vi "ref_MCListbox_call.vi"(8 "VI引用输入":refnum<vi>, 9 "清除原有数据":bool, 10 "数组":string[][](array[string])) -> ()   [LabVIEW 2016]
uses:
  <vilib>/Utility/miscctls.llb/LVRowAndColumnTypeDef.ctl
  Global Variables/Pacemaker ASIC Test_Save_SN Globals.vi
  Global Variables/Pacemaker ASIC Test_Config Globals.vi
  <vilib>/Utility/file.llb/Write Delimited Spreadsheet (string).vi
panel:
  out "数组 2":string[](array[string])
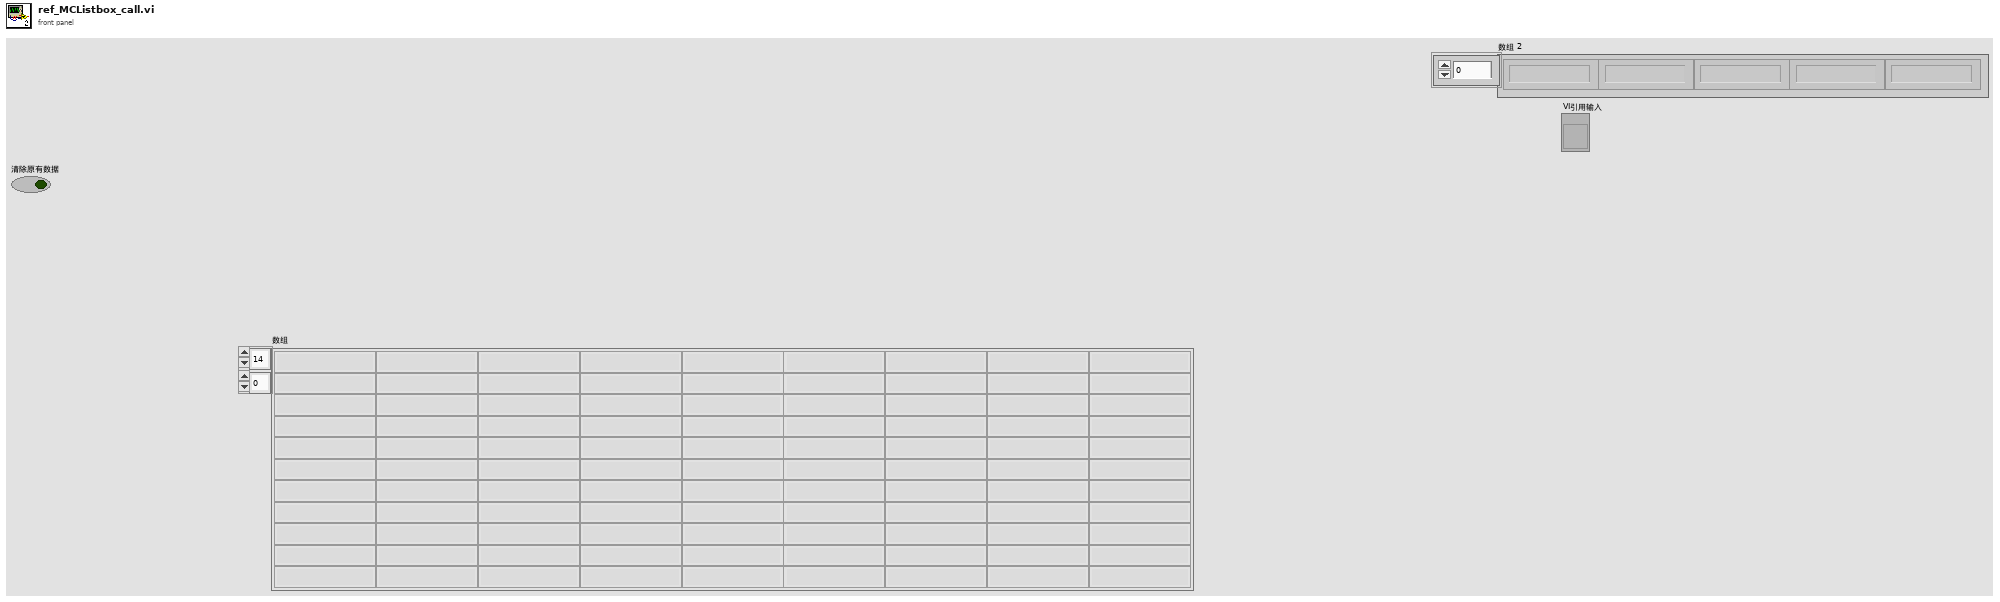
[diagram p1: front panel]
types:
  T1 = cluster{"LED1":refnum<vi>, "LED2":refnum<vi>, "LED3":refnum<vi>, "LED4":refnum<vi>, "LED5":refnum<vi>, "LED7":refnum<vi>, "LED8":refnum<vi>, "LED9":refnum<vi>, "LED10":refnum<vi>}
  T2 = typedef "LVRowAndColumnTypeDef.ctl" = cluster{"Row":i32, "Column":i32}
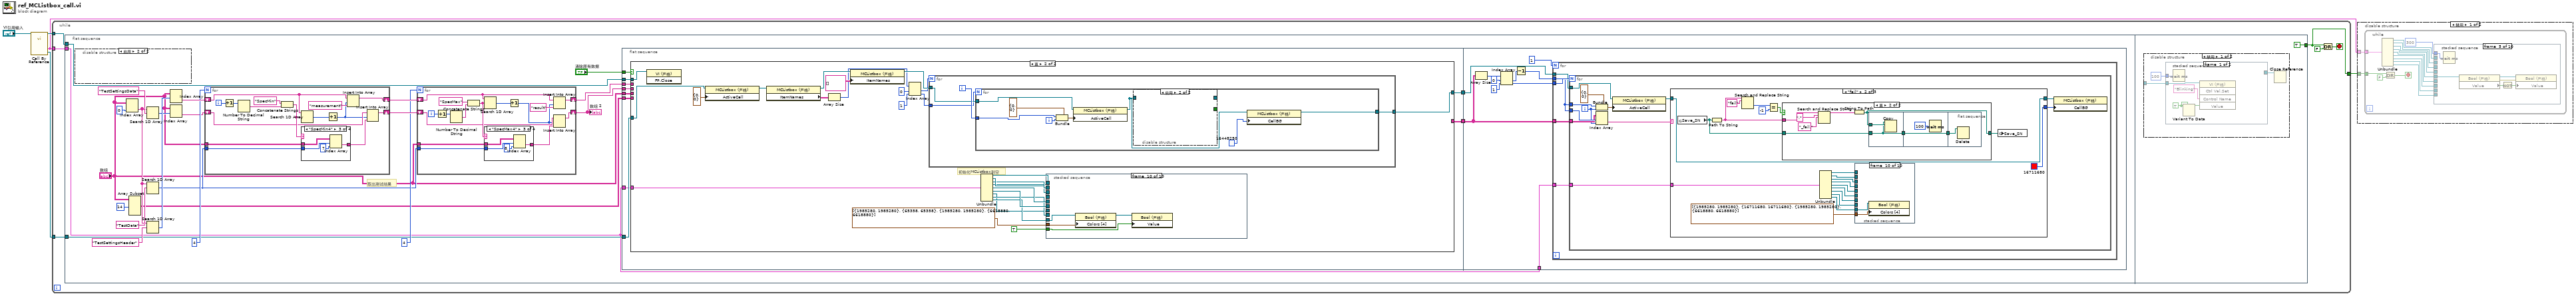
[diagram p0: block diagram]
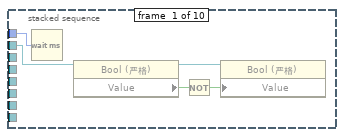
[diagram p2: hidden frame]
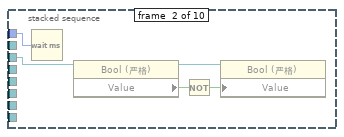
[diagram p3: hidden frame]
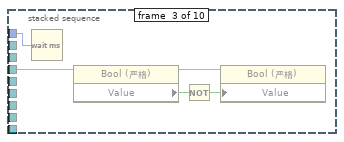
[diagram p4: hidden frame]
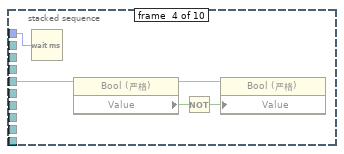
[diagram p5: hidden frame]
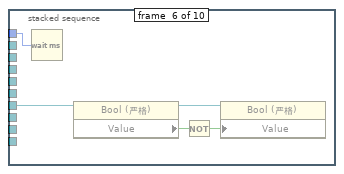
[diagram p6: hidden frame]
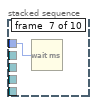
[diagram p7: hidden frame]
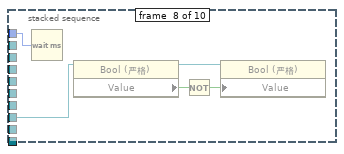
[diagram p8: hidden frame]
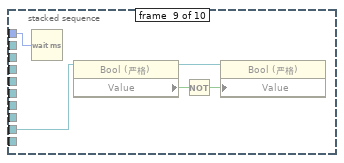
[diagram p9: hidden frame]
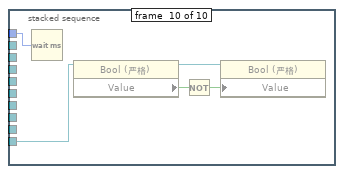
[diagram p10: hidden frame]
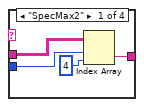
[diagram p12: hidden frame]
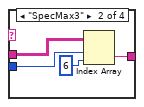
[diagram p13: hidden frame]
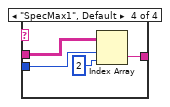
[diagram p14: hidden frame]
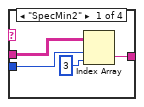
[diagram p15: hidden frame]
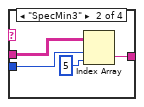
[diagram p16: hidden frame]
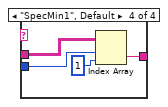
[diagram p17: hidden frame]
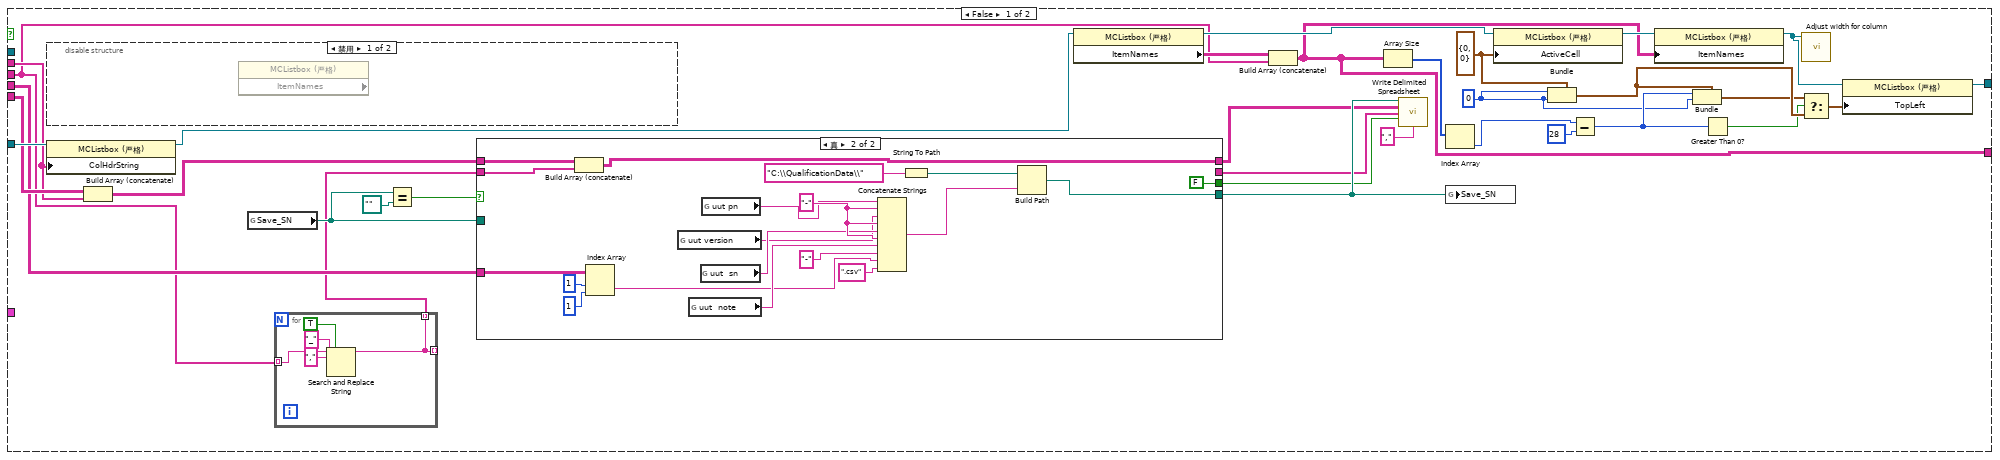
[diagram p18: hidden frame]
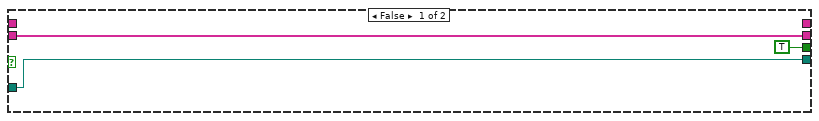
[diagram p20: hidden frame]
diagram:
  n1 = call-by-ref "?"(reference="VI引用输入") -> (reference out=w4:refnum<vi>, "引用输出"=w3:refnum<vi>, "输出簇"=w1:T1)  [unwired: 11 in, 1 out]
  n2 = while {
    tunnel: w4 -> [w11]
    tunnel: w3 -> [w10]
    tunnel: [w7] -> w2
    tunnel: w1 -> [w6]
    stop <- w8 stop-if-true
    n3 = flat-sequence {
      tunnel: w11 -> [w16]
      tunnel: w10 -> [w17]
      tunnel: w6 -> [w15]
      tunnel: [TRUE] -> w7
      frame #0 {
        # "取出测试结果"
        n4 = disable-structure shown="启用" {
          frame Disabled {
            n5 = Index Array(index (col)=0 ("禁用的索引 (列)")) -> (element=w337)  [unwired: 2 in]
            n6 = Search 1D Array(1D array=w337, element="" ("元素")) -> (index of element=w340:i32)  [unwired: 1 in]
            n7 = Bundle(cluster=T2 {"Row"=0, "Column"=0} ("活动单元格:活动单元格"), "Row"=w340, "Column"=0 ("元素")) -> ()  [unwired: 1 out]
          }
          frame Enabled {
          }
        }
        n8 = Index Array(array="数组", index (col)=0 ("禁用的索引 (列)")) -> (element=w20:string[])  [unwired: 1 in]
        n9 = Array Subset(array="数组", length (row)=14 ("长度")) -> (w13:string[][])  [unwired: 3 in]
        n10 = Search 1D Array(1D array=w20, element="TestSettingsData" ("元素")) -> (index of element=w21:i32)  [unwired: 1 in]
        n11 = Search 1D Array(1D array=w20, element="TestData" ("元素")) -> (index of element=w18:i32)  [unwired: 1 in]
        n12 = Search 1D Array(1D array=w20, element="TestSettingsHeader" ("元素")) -> (index of element=w23:i32)  [unwired: 1 in]
        n13 = Index Array(array="数组", index (row)=w23) -> (element=w34:string[])  [unwired: 1 in]
        n14 = Index Array(array="数组", index (row)=w21) -> (element=w32:string[])  [unwired: 1 in]
        n15 = for {
          N: 4 -> [_]
          shift-right: [w76] -> w31
          shift-left: w34 -> [w77]
          shift-right: [w73] -> w30
          shift-left: w32 -> [w74]
          tunnel: "数组" -> [w69]
          tunnel: w18 -> [w68]
          i -> [w81]
          n16 = Increment(x=w81) -> (x+1=w80:i32)
          n17 = Number To Decimal String(number=w80) -> (decimal integer string=w79:string)  [unwired: 1 in]
          n18 = Concatenate Strings("SpecMin" ("元素"), w79) -> (w78:string)
          n19 = Search 1D Array(1D array=w77, element=w78) -> (index of element=w75:i32)  [unwired: 1 in]
          n20 = case shown="\"SpecMin4\"" w78 {
            tunnel: w69 -> [w85 w89 w91 w98]
            tunnel: [w84 w87 w93 w96] -> w71
            tunnel: w68 -> [w83 w88 w92 w95]
            frame "SpecMin2" {
              n21 = Index Array(array=w85, index (row)=w83, index (col)=3) -> (element=w84:string)
            }
            frame "SpecMin3" {
              n22 = Index Array(array=w89, index (row)=w88, index (col)=5) -> (element=w87:string)
            }
            frame "SpecMin4" {
              n23 = Index Array(array=w91, index (row)=w92, index (col)=7) -> (element=w93:string)
            }
            frame "SpecMin1", Default {
              n24 = Index Array(array=w98, index (row)=w95, index (col)=1) -> (element=w96:string)
            }
          }
          n25 = Increment(x=w75) -> (x+1=w70:i32)
          n26 = Insert Into Array(array=w77, index=w70, new element="measurement" ("新元素/子数组")) -> (w76:string[])
          n27 = Insert Into Array(array=w74, index=w70, new element=w71) -> (w73:string[])
        }
        n28 = for {
          N: 4 -> [_]
          shift-right: [w45] -> w28
          shift-left: w31 -> [w46]
          shift-right: [w42] -> w27
          shift-left: w30 -> [w43]
          tunnel: "数组" -> [w38]
          tunnel: w18 -> [w37]
          i -> [w50]
          n29 = Increment(x=w50) -> (x+1=w49:i32)
          n30 = Number To Decimal String(number=w49) -> (decimal integer string=w48:string)  [unwired: 1 in]
          n31 = Concatenate Strings("SpecMax" ("元素"), w48) -> (w47:string)
          n32 = Search 1D Array(1D array=w46, element=w47) -> (index of element=w44:i32)  [unwired: 1 in]
          n33 = case shown="\"SpecMax4\"" w47 {
            tunnel: w38 -> [w54 w58 w61 w67]
            tunnel: [w53 w56 w62 w65] -> w40
            tunnel: w37 -> [w52 w57 w60 w64]
            frame "SpecMax2" {
              n34 = Index Array(array=w54, index (row)=w52, index (col)=4) -> (element=w53:string)
            }
            frame "SpecMax3" {
              n35 = Index Array(array=w58, index (row)=w57, index (col)=6) -> (element=w56:string)
            }
            frame "SpecMax4" {
              n36 = Index Array(array=w61, index (row)=w60, index (col)=8) -> (element=w62:string)
            }
            frame "SpecMax1", Default {
              n37 = Index Array(array=w67, index (row)=w64, index (col)=2) -> (element=w65:string)
            }
          }
          n38 = Increment(x=w44) -> (x+1=w39:i32)
          n39 = Insert Into Array(array=w46, index=w39, new element="result" ("新元素/子数组")) -> (w45:string[])
          n40 = Insert Into Array(array=w43, index=w39, new element=w40) -> (w42:string[])
        }
        "数组 2" <- w27
        n41 = flat-sequence {
          tunnel: w28 -> [w108]
          tunnel: w27 -> [w107]
          tunnel: "清除原有数据" -> [w106]
          tunnel: w17 -> [w105]
          tunnel: [w104] -> w36
          tunnel: [w103] -> w35
          tunnel: w16 -> [w102]
          tunnel: w15 -> [w101]
          tunnel: w13 -> [w100]
          tunnel: "数组" -> [w99]
          tunnel: w36 -> [w256]
          tunnel: w35 -> [w255]
          tunnel: w15 -> [w254]
          frame #0 {
            n42 = case shown="真" w106 {
              tunnel: w108 -> [w133 _]
              tunnel: w107 -> [w111 _]
              tunnel: w105 -> [w137 w192]
              tunnel: [w124 _] -> w104
              tunnel: [w118 w189] -> w103
              tunnel: w102 -> [_ w191]
              tunnel: w101 -> [_ w188]
              tunnel: w100 -> [w134 _]
              tunnel: w99 -> [w132 _]
              frame False {
                w112 = 0
                w122 = T2 {"Row"=0, "Column"=0} ("活动单元格:活动单元格")
                n43 = disable-structure shown="禁用" {
                  frame Disabled {
                    n44 = property class="MCListbox (严格)"() -> ("ItemNames"=w146:string[][])  [unwired: 2 in, 2 out]
                  }
                  frame Enabled {
                  }
                }
                n45 = property class="MCListbox (严格)"(reference=w137, "ColHdrString"=w133) -> (reference out=w136:refnum<vi>)  [unwired: 1 in, 1 out]
                n46 = Build Array (concatenate)(w134, w133) -> (w135:string[][])
                n47 = global read "Pacemaker ASIC Test_Save_SN Globals.vi" "Save_SN"() -> (w129:path)
                n48 = for {
                  tunnel: w111 -> [w145] mode=indexing
                  tunnel: [w142] -> _ mode=indexing
                  tunnel: [w142] -> w110 mode=indexing
                  n49 = Search and Replace String(replace all?=TRUE ("替换全部？(F)"), input string=w145, search string="," ("搜索字符串"), replace string="_" ("替换字符串(\"\")")) -> (result string=w142:string)  [unwired: 4 in, 3 out]
                }
                n50 = Equal?(x=w129, y=path "") -> (x = y?=w130:bool)
                n51 = case shown="真" w130 {
                  tunnel: w135 -> [_ w152]
                  tunnel: w132 -> [_ w156]
                  tunnel: w129 -> [w149 _]
                  tunnel: [w149 w154] -> w128
                  tunnel: [_ w150] -> w127
                  tunnel: [TRUE FALSE] -> w126
                  tunnel: w110 -> [w147 w151]
                  tunnel: [w147 _] -> w125
                  frame False {
                  }
                  frame True {
                    w167 = "-"
                    n52 = Build Array (concatenate)(w152, w151) -> (w150:string[][])
                    n53 = Index Array(array=w156, index (row)=1 ("索引 (行)"), index (col)=1 ("禁用的索引 (列)")) -> (element=w155:string)
                    n54 = global read "Pacemaker ASIC Test_Config Globals.vi" "uut version"() -> (w165:string)
                    n55 = global read "Pacemaker ASIC Test_Config Globals.vi" "uut  note"() -> (w168:string)
                    n56 = global read "Pacemaker ASIC Test_Config Globals.vi" "uut  sn"() -> (w166:string)
                    n57 = global read "Pacemaker ASIC Test_Config Globals.vi" "uut pn"() -> (w164:string)
                    n58 = Concatenate Strings(w164, w167, w165, w167, w166, w167, w168, "-", w155, ".csv" ("字符串")) -> (w160:string)
                    n59 = String To Path(string="C:\\QualificationData\\" ("字符串")) -> (path=w161:path)
                    n60 = Build Path(base path=w161, name or relative path=w160) -> (appended path=w154:path)
                  }
                }
                n61 = property class="MCListbox (严格)"(reference=w136) -> (reference out=w138:refnum<vi>, "ItemNames"=w139:string[][])  [unwired: 1 in, 1 out]
                n62 = Build Array (concatenate)(w139, w111) -> (w124:string[][])
                n63 = Array Size(array=w124) -> (size(s)=w123:i32[])
                n64 = call-poly <vilib>:"Write Delimited Spreadsheet.vi"("file path (dialog if empty)"=w128, "2D data"=w127, "1D data"=w125, "append to file? (new file:F)"=w126, "delimiter (\\t)"="," ("delimiter (\\t)")) -> ()  [unwired: 9 in, 2 out]
                n65 = Index Array(array=w123) -> (element=w116:i32)  [unwired: 1 in]
                n66 = global write "Pacemaker ASIC Test_Save_SN Globals.vi" "Save_SN"(w128) -> ()
                n67 = property class="MCListbox (严格)"(reference=w138, "ActiveCell"=w122) -> (reference out=w140:refnum<vi>)  [unwired: 1 in, 1 out]
                n68 = Bundle(cluster=w122, "Row"=w112, "Column"=w112) -> (w121:T2)
                n69 = Subtract(x=w116, y=28) -> (x-y=w113:i32)
                n70 = property class="MCListbox (严格)"(reference=w140, "ItemNames"=w124) -> (reference out=w117:refnum<vi>)  [unwired: 1 in, 1 out]
                n71 = Bundle(cluster=w121, "Row"=w113, "Column"=w112) -> (w120:T2)
                n72 = Greater Than 0?(x=w113) -> (x > 0?=w114:bool)
                n73 = call "Adjust width for column.vi"("MCListbox引用句柄"=w117) -> ()  [unwired: 11 in]
                n74 = Select(t=w120, s=w114, f=w121) -> (s? t:f=w119:T2)
                n75 = property class="MCListbox (严格)"(reference=w117, "TopLeft"=w119) -> (reference out=w118:refnum<vi>)  [unwired: 1 in, 1 out]
              }
              frame True {
                # "初始化MCListbox到空"
                n76 = invoke class="VI (严格)" method="FP.Close"(reference=w191) -> ()  [unwired: 2 in, 3 out]
                n77 = property class="MCListbox (严格)"(reference=w192, "ActiveCell"=T2 {"Row"=0, "Column"=0} ("活动单元格:活动单元格")) -> (reference out=w176:refnum<vi>)  [unwired: 1 in, 1 out]
                n78 = property class="MCListbox (严格)"(reference=w176) -> (reference out=w175:refnum<vi>, "ItemNames"=w174:string[][])  [unwired: 1 in, 1 out]
                n79 = Array Size(array=w174) -> (size(s)=w173:i32[])
                n80 = property class="MCListbox (严格)"(reference=w175, "ItemNames"=string[][] [] ("项名")) -> (reference out=w190:refnum<vi>)  [unwired: 1 in, 1 out]
                n81 = Index Array(array=w173, index #1=0 ("索引"), index #2=1 ("索引")) -> (element #1=w171:i32, element #2=w169:i32)
                n82 = for {
                  N: w171 -> [_]
                  tunnel: w190 -> [w237]
                  tunnel: [w236] -> w189
                  tunnel: w169 -> [w235]
                  i -> [w238]
                  n83 = for {
                    N: w235 -> [_]
                    tunnel: w238 -> [w245]
                    tunnel: w237 -> [w242]
                    tunnel: [w241] -> w236
                    i -> [w244]
                    n84 = Bundle(cluster=cluster{i32, i32} {0, 0} ("簇"), w245, w244) -> (w246:cluster{i32, i32})
                    n85 = property class="MCListbox (严格)"(reference=w242, "ActiveCell"=w246) -> (reference out=w239:refnum<vi>)  [unwired: 1 in, 1 out]
                    n86 = disable-structure shown="启用" {
                      disable-tunnel: w239 -> [w249 _]
                      disable-tunnel: [w248 _] -> _
                      disable-tunnel: [w247 _] -> _
                      frame Disabled {
                        n87 = property class="MCListbox (严格)"(reference=w249) -> (reference out=w248:refnum<vi>, "CellBG"=w250:u32)  [unwired: 1 in, 1 out]
                        n88 = Not Equal?(x=w250) -> (x != y?=w247:bool)  [unwired: 1 in]
                      }
                      frame Enabled {
                      }
                    }
                    n89 = property class="MCListbox (严格)"(reference=w239, "CellBG"=u32 16448250) -> (reference out=w241:refnum<vi>)  [unwired: 1 in, 1 out]
                  }
                }
                n90 = Unbundle(w188) -> ("LED1"=w187:refnum<vi>, "LED2"=w186:refnum<vi>, "LED3"=w185:refnum<vi>, "LED4"=w184:refnum<vi>, "LED5"=w183:refnum<vi>, "LED7"=w182:refnum<vi>, "LED8"=w179:refnum<vi>, "LED9"=w180:refnum<vi>, "LED10"=w181:refnum<vi>)
                n91 = stacked-sequence {
                  tunnel: w187 -> [w198 _ _ _ _ _ _ _ _ _]
                  tunnel: w186 -> [_ w202 _ _ _ _ _ _ _ _]
                  tunnel: w185 -> [_ _ w206 _ _ _ _ _ _ _]
                  tunnel: w184 -> [_ _ _ w210 _ _ _ _ _ _]
                  tunnel: w183 -> [_ _ _ _ w214 _ _ _ _ _]
                  tunnel: w182 -> [_ _ _ _ _ w218 _ _ _ _]
                  tunnel: w181 -> [_ _ _ _ _ _ _ _ _ w234]
                  tunnel: w180 -> [_ _ _ _ _ _ _ _ w229 _]
                  tunnel: w179 -> [_ _ _ _ _ _ w222 w226 _ _]
                  tunnel: cluster{u32, u32}[] [{1985280, 1985280}, {65358, 65358}, {1985280, 1985280}, {6618880, 6618880}] ("颜色[4]") -> [w197 w201 w205 w209 w213 w217 w221 w225 w230 w233]
                  tunnel: TRUE -> [w196 w200 w204 w207 w211 w215 w219 w223 w227 w231]
                  frame #0 {
                    n92 = property class="Bool (严格)"(reference=w198, "Colors [4]"=w197) -> (reference out=w195:refnum<vi>)  [unwired: 1 in, 1 out]
                    n93 = property class="Bool (严格)"(reference=w195, "Value"=w196) -> ()  [unwired: 1 in, 2 out]
                  }
                  frame #1 {
                    n94 = property class="Bool (严格)"(reference=w202, "Colors [4]"=w201) -> (reference out=w199:refnum<vi>)  [unwired: 1 in, 1 out]
                    n95 = property class="Bool (严格)"(reference=w199, "Value"=w200) -> ()  [unwired: 1 in, 2 out]
                  }
                  frame #2 {
                    n96 = property class="Bool (严格)"(reference=w206, "Colors [4]"=w205) -> (reference out=w203:refnum<vi>)  [unwired: 1 in, 1 out]
                    n97 = property class="Bool (严格)"(reference=w203, "Value"=w204) -> ()  [unwired: 1 in, 2 out]
                  }
                  frame #3 {
                    n98 = property class="Bool (严格)"(reference=w210, "Colors [4]"=w209) -> (reference out=w208:refnum<vi>)  [unwired: 1 in, 1 out]
                    n99 = property class="Bool (严格)"(reference=w208, "Value"=w207) -> ()  [unwired: 1 in, 2 out]
                  }
                  frame #4 {
                    n100 = property class="Bool (严格)"(reference=w214, "Colors [4]"=w213) -> (reference out=w212:refnum<vi>)  [unwired: 1 in, 1 out]
                    n101 = property class="Bool (严格)"(reference=w212, "Value"=w211) -> ()  [unwired: 1 in, 2 out]
                  }
                  frame #5 {
                    n102 = property class="Bool (严格)"(reference=w218, "Colors [4]"=w217) -> (reference out=w216:refnum<vi>)  [unwired: 1 in, 1 out]
                    n103 = property class="Bool (严格)"(reference=w216, "Value"=w215) -> ()  [unwired: 1 in, 2 out]
                  }
                  frame #6 {
                    n104 = property class="Bool (严格)"(reference=w222, "Colors [4]"=w221) -> (reference out=w220:refnum<vi>)  [unwired: 1 in, 1 out]
                    n105 = property class="Bool (严格)"(reference=w220, "Value"=w219) -> ()  [unwired: 1 in, 2 out]
                  }
                  frame #7 {
                    n106 = property class="Bool (严格)"(reference=w226, "Colors [4]"=w225) -> (reference out=w224:refnum<vi>)  [unwired: 1 in, 1 out]
                    n107 = property class="Bool (严格)"(reference=w224, "Value"=w223) -> ()  [unwired: 1 in, 2 out]
                  }
                  frame #8 {
                    n108 = property class="Bool (严格)"(reference=w229, "Colors [4]"=w230) -> (reference out=w228:refnum<vi>)  [unwired: 1 in, 1 out]
                    n109 = property class="Bool (严格)"(reference=w228, "Value"=w227) -> ()  [unwired: 1 in, 2 out]
                  }
                  frame #9 {
                    n110 = property class="Bool (严格)"(reference=w234, "Colors [4]"=w233) -> (reference out=w232:refnum<vi>)  [unwired: 1 in, 1 out]
                    n111 = property class="Bool (严格)"(reference=w232, "Value"=w231) -> ()  [unwired: 1 in, 2 out]
                  }
                }
              }
            }
          }
          frame #1 {
            n112 = Array Size(array=w256) -> (size(s)=w260:i32[])
            n113 = Index Array(array=w260, index #1=0 ("索引"), index #2=1 ("索引")) -> (element #1=w253:i32, element #2=w257:i32)
            n114 = Decrement(x=w253) -> (x-1=w252:i32)
            n115 = for {
              N: 1 -> [_]
              tunnel: w257 -> [w265]
              tunnel: w256 -> [w264]
              tunnel: w255 -> [w263]
              tunnel: w254 -> [w262]
              tunnel: w252 -> [w261]
              n116 = for {
                N: w265 -> [_]
                tunnel: w261 -> [w277]
                tunnel: w264 -> [w276]
                tunnel: w261 -> [w273]
                tunnel: w263 -> [w267]
                tunnel: w262 -> [w266]
                i -> [w272]
                n117 = Bundle(cluster=cluster{i32, i32} {0, 0} ("簇"), w273, w272) -> (w274:cluster{i32, i32})
                n118 = Index Array(array=w276, index (row)=w277, index (col)=w272) -> (element=w275:string)
                n119 = property class="MCListbox (严格)"(reference=w267, "ActiveCell"=w274) -> (reference out=w271:refnum<vi>)  [unwired: 1 in, 1 out]
                n120 = case shown="\"fail\"" w275 {
                  tunnel: w271 -> [w279 w299 w335]
                  tunnel: [w279 w299 w335] -> w270
                  tunnel: [u32 6618880 u32 16711680 u32 16448250] -> w268
                  tunnel: w266 -> [_ w288 _]
                  frame "pass" {
                  }
                  frame "fail" {
                    n121 = global read "Pacemaker ASIC Test_Save_SN Globals.vi" "Save_SN"() -> (w280:path)
                    n122 = Path To String(path=w280) -> (string=w282:string)
                    n123 = Search and Replace String(input string=w282, search string="fail" ("搜索字符串")) -> (offset past replacement=w285:i32)  [unwired: 6 in, 3 out]
                    n124 = Equal?(x=w285, y=-1) -> (x = y?=w283:bool)
                    n125 = case shown="真" w283 {
                      tunnel: w282 -> [_ w304]
                      tunnel: [w300 w307] -> w281
                      tunnel: w280 -> [w300 w308]
                      frame False {
                      }
                      frame True {
                        n126 = Search and Replace String(input string=w304, search string="." ("搜索字符串"), replace string="_fail." ("字符串")) -> (result string=w301:string)  [unwired: 5 in, 3 out]
                        n127 = String To Path(string=w301) -> (path=w307:path)
                        n128 = flat-sequence {
                          tunnel: w308 -> [w309]
                          tunnel: w307 -> [w310]
                          tunnel: [w309] -> w305
                          tunnel: [w311] -> w306
                          tunnel: w305 -> [w311]
                          tunnel: w306 -> [w313]
                          frame #0 {
                            n129 = Copy(10:w310, 11:w309) -> ()  [unwired: 3 in, 3 out]
                          }
                          frame #1 {
                            n130 = Wait (ms)(milliseconds to wait=u32 100 ("等待时间（毫秒）")) -> ()  [unwired: 1 out]
                          }
                          frame #2 {
                            n131 = Delete(path (use dialog)=w313) -> ()  [unwired: 4 in, 3 out]
                          }
                        }
                      }
                    }
                    n132 = Unbundle(w288) -> ("LED1"=w297:refnum<vi>, "LED2"=w296:refnum<vi>, "LED3"=w295:refnum<vi>, "LED4"=w294:refnum<vi>, "LED5"=w293:refnum<vi>, "LED7"=w292:refnum<vi>, "LED8"=w289:refnum<vi>, "LED9"=w290:refnum<vi>, "LED10"=w291:refnum<vi>)
                    n133 = stacked-sequence {
                      tunnel: w297 -> [w315 _ _ _ _ _ _ _ _ _]
                      tunnel: w296 -> [_ w317 _ _ _ _ _ _ _ _]
                      tunnel: w295 -> [_ _ w319 _ _ _ _ _ _ _]
                      tunnel: w294 -> [_ _ _ w321 _ _ _ _ _ _]
                      tunnel: w293 -> [_ _ _ _ w323 _ _ _ _ _]
                      tunnel: w292 -> [_ _ _ _ _ w325 _ _ _ _]
                      tunnel: w291 -> [_ _ _ _ _ _ _ _ _ w333]
                      tunnel: w290 -> [_ _ _ _ _ _ _ _ w330 _]
                      tunnel: w289 -> [_ _ _ _ _ _ w327 w329 _ _]
                      tunnel: cluster{u32, u32}[] [{1985280, 1985280}, {16711680, 16711680}, {1985280, 1985280}, {6618880, 6618880}] ("颜色[4]") -> [w314 w316 w318 w320 w322 w324 w326 w328 w331 w332]
                      frame #0 {
                        n134 = property class="Bool (严格)"(reference=w315, "Colors [4]"=w314) -> ()  [unwired: 1 in, 2 out]
                      }
                      frame #1 {
                        n135 = property class="Bool (严格)"(reference=w317, "Colors [4]"=w316) -> ()  [unwired: 1 in, 2 out]
                      }
                      frame #2 {
                        n136 = property class="Bool (严格)"(reference=w319, "Colors [4]"=w318) -> ()  [unwired: 1 in, 2 out]
                      }
                      frame #3 {
                        n137 = property class="Bool (严格)"(reference=w321, "Colors [4]"=w320) -> ()  [unwired: 1 in, 2 out]
                      }
                      frame #4 {
                        n138 = property class="Bool (严格)"(reference=w323, "Colors [4]"=w322) -> ()  [unwired: 1 in, 2 out]
                      }
                      frame #5 {
                        n139 = property class="Bool (严格)"(reference=w325, "Colors [4]"=w324) -> ()  [unwired: 1 in, 2 out]
                      }
                      frame #6 {
                        n140 = property class="Bool (严格)"(reference=w327, "Colors [4]"=w326) -> ()  [unwired: 1 in, 2 out]
                      }
                      frame #7 {
                        n141 = property class="Bool (严格)"(reference=w329, "Colors [4]"=w328) -> ()  [unwired: 1 in, 2 out]
                      }
                      frame #8 {
                        n142 = property class="Bool (严格)"(reference=w330, "Colors [4]"=w331) -> ()  [unwired: 1 in, 2 out]
                      }
                      frame #9 {
                        n143 = property class="Bool (严格)"(reference=w333, "Colors [4]"=w332) -> ()  [unwired: 1 in, 2 out]
                      }
                    }
                    n144 = global write "Pacemaker ASIC Test_Save_SN Globals.vi" "Save_SN"(w281) -> ()
                  }
                  frame Default {
                  }
                }
                n145 = property class="MCListbox (严格)"(reference=w270, "CellBG"=w268) -> ()  [unwired: 1 in, 2 out]
              }
            }
          }
        }
      }
      frame #1 {
        n146 = disable-structure shown="禁用" {
          disable-tunnel: _ -> [w343 _]
          frame Disabled {
            n147 = stacked-sequence {
              tunnel: w343 -> [w349 w355]
              tunnel: 100 -> [w346 w352]
              tunnel: [_ w351] -> w344
              frame #0 {
                w348 = TRUE
                n148 = Wait (ms)(milliseconds to wait=w346) -> ()  [unwired: 1 out]
                n149 = Variant To Data(type=w348, Variant=w348) -> (data=w347:bool)  [unwired: 1 in, 1 out]
                n150 = invoke class="VI (严格)" method="Ctrl Val.Set"(reference=w349, "Control Name"="Blinking" ("控件名"), "Value"=w347) -> ()  [unwired: 2 in, 5 out]
              }
              frame #1 {
                w354 = FALSE
                n151 = Wait (ms)(milliseconds to wait=w352) -> ()  [unwired: 1 out]
                n152 = Variant To Data(type=w354, Variant=w354) -> (data=w353:bool)  [unwired: 1 in, 1 out]
                n153 = invoke class="VI (严格)" method="Ctrl Val.Set"(reference=w355, "Control Name"="Blinking" ("控件名"), "Value"=w353) -> (reference out=w351:refnum<vi>)  [unwired: 2 in, 4 out]
              }
            }
            n154 = Close Reference(reference=w344) -> ()  [unwired: 1 in, 1 out]
          }
          frame Enabled {
          }
        }
      }
    }
    n155 = Or(x=w7, y=FALSE) -> (x .or. y?=w8:bool)
  }
  n156 = disable-structure shown="禁用" {
    disable-tunnel: w2 -> [w358 _]
    disable-tunnel: w1 -> [w357 _]
    frame Disabled {
      n157 = while {
        tunnel: w357 -> [w372]
        tunnel: w358 -> [w361]
        stop <- w360 stop-if-true
        n158 = Unbundle(w372) -> ("LED1"=w371:refnum<vi>, "LED2"=w369:refnum<vi>, "LED3"=w368:refnum<vi>, "LED4"=w367:refnum<vi>, "LED5"=w366:refnum<vi>, "LED7"=w365:refnum<vi>, "LED8"=w362:refnum<vi>, "LED9"=w363:refnum<vi>, "LED10"=w364:refnum<vi>)
        n159 = Or(x=w361, y=FALSE) -> (x .or. y?=w360:bool)
        n160 = stacked-sequence {
          tunnel: w371 -> [w377 _ _ _ _ _ _ _ _ _]
          tunnel: 300 -> [w373 w380 w383 w388 w394 w401 w404 w407 w410 w417]
          tunnel: w369 -> [_ w382 _ _ _ _ _ _ _ _]
          tunnel: w368 -> [_ _ w384 _ _ _ _ _ _ _]
          tunnel: w367 -> [_ _ _ w392 _ _ _ _ _ _]
          tunnel: w366 -> [_ _ _ _ w393 _ _ _ _ _]
          tunnel: w365 -> [_ _ _ _ _ w400 _ _ _ _]
          tunnel: w364 -> [_ _ _ _ _ _ _ _ _ w419]
          tunnel: w363 -> [_ _ _ _ _ _ _ _ w414 _]
          tunnel: w362 -> [_ _ _ _ _ _ _ w409 _ _]
          frame #0 {
            n161 = Wait (ms)(milliseconds to wait=w373) -> ()  [unwired: 1 out]
            n162 = property class="Bool (严格)"(reference=w377) -> (reference out=w376:refnum<vi>, "Value"=w375:bool)  [unwired: 1 in, 1 out]
            n163 = Not(x=w375) -> (.not. x?=w374:bool)
            n164 = property class="Bool (严格)"(reference=w376, "Value"=w374) -> ()  [unwired: 1 in, 2 out]
          }
          frame #1 {
            n165 = Wait (ms)(milliseconds to wait=w380) -> ()  [unwired: 1 out]
            n166 = property class="Bool (严格)"(reference=w382) -> (reference out=w381:refnum<vi>, "Value"=w379:bool)  [unwired: 1 in, 1 out]
            n167 = Not(x=w379) -> (.not. x?=w378:bool)
            n168 = property class="Bool (严格)"(reference=w381, "Value"=w378) -> ()  [unwired: 1 in, 2 out]
          }
          frame #2 {
            n169 = Wait (ms)(milliseconds to wait=w383) -> ()  [unwired: 1 out]
            n170 = property class="Bool (严格)"(reference=w384) -> (reference out=w385:refnum<vi>, "Value"=w387:bool)  [unwired: 1 in, 1 out]
            n171 = Not(x=w387) -> (.not. x?=w386:bool)
            n172 = property class="Bool (严格)"(reference=w385, "Value"=w386) -> ()  [unwired: 1 in, 2 out]
          }
          frame #3 {
            n173 = Wait (ms)(milliseconds to wait=w388) -> ()  [unwired: 1 out]
            n174 = property class="Bool (严格)"(reference=w392) -> (reference out=w391:refnum<vi>, "Value"=w390:bool)  [unwired: 1 in, 1 out]
            n175 = Not(x=w390) -> (.not. x?=w389:bool)
            n176 = property class="Bool (严格)"(reference=w391, "Value"=w389) -> ()  [unwired: 1 in, 2 out]
          }
          frame #4 {
            n177 = Wait (ms)(milliseconds to wait=w394) -> ()  [unwired: 1 out]
            n178 = property class="Bool (严格)"(reference=w393) -> (reference out=w398:refnum<vi>, error out=w397:errorcluster, "Value"=w396:bool)  [unwired: 1 in]
            n179 = Not(x=w396) -> (.not. x?=w395:bool)
            n180 = property class="Bool (严格)"(reference=w398, error in=w397, "Value"=w395) -> ()  [unwired: 2 out]
          }
          frame #5 {
            n181 = Wait (ms)(milliseconds to wait=w401) -> ()  [unwired: 1 out]
            n182 = property class="Bool (严格)"(reference=w400) -> (reference out=w399:refnum<vi>, "Value"=w403:bool)  [unwired: 1 in, 1 out]
            n183 = Not(x=w403) -> (.not. x?=w402:bool)
            n184 = property class="Bool (严格)"(reference=w399, "Value"=w402) -> ()  [unwired: 1 in, 2 out]
          }
          frame #6 {
            n185 = Wait (ms)(milliseconds to wait=w404) -> ()  [unwired: 1 out]
          }
          frame #7 {
            n186 = Wait (ms)(milliseconds to wait=w407) -> ()  [unwired: 1 out]
            n187 = property class="Bool (严格)"(reference=w409) -> (reference out=w408:refnum<vi>, "Value"=w406:bool)  [unwired: 1 in, 1 out]
            n188 = Not(x=w406) -> (.not. x?=w405:bool)
            n189 = property class="Bool (严格)"(reference=w408, "Value"=w405) -> ()  [unwired: 1 in, 2 out]
          }
          frame #8 {
            n190 = Wait (ms)(milliseconds to wait=w410) -> ()  [unwired: 1 out]
            n191 = property class="Bool (严格)"(reference=w414) -> (reference out=w413:refnum<vi>, "Value"=w412:bool)  [unwired: 1 in, 1 out]
            n192 = Not(x=w412) -> (.not. x?=w411:bool)
            n193 = property class="Bool (严格)"(reference=w413, "Value"=w411) -> ()  [unwired: 1 in, 2 out]
          }
          frame #9 {
            n194 = Wait (ms)(milliseconds to wait=w417) -> ()  [unwired: 1 out]
            n195 = property class="Bool (严格)"(reference=w419) -> (reference out=w418:refnum<vi>, "Value"=w416:bool)  [unwired: 1 in, 1 out]
            n196 = Not(x=w416) -> (.not. x?=w415:bool)
            n197 = property class="Bool (严格)"(reference=w418, "Value"=w415) -> ()  [unwired: 1 in, 2 out]
          }
        }
      }
    }
    frame Enabled {
    }
  }
